vi "FTW-Test-JSON-TypeCoerce-Numbers.vi"() -> (0 "Test Result":errorcluster)   [LabVIEW 2015]
uses:
  src/json/FTW-JSON-Type.ctl
  src/json/core/FTW-JSON-Core-Type.ctl
  src/reflection/FTW-Reflection-Types.ctl
  lib/FTW-KernelFilepath.vi
  codegen/xnode/json/fetch/FTW-JSON-Core-GetFlattenedValue.vi
  src/json/core/FTW-JSON-Core-LibraryReturnValue.vi
  src/error/FTW-ERR-ThrowInvalidReferenceError.vi
  src/json/core/FTW-JSON-Core-ElementType.vi
  codegen/xnode/FTW-JSON-Fetch.xnode
  src/core/type/FTW-Type-JSON.ctl
panel:
  out "JSON String (UTF-8)":string
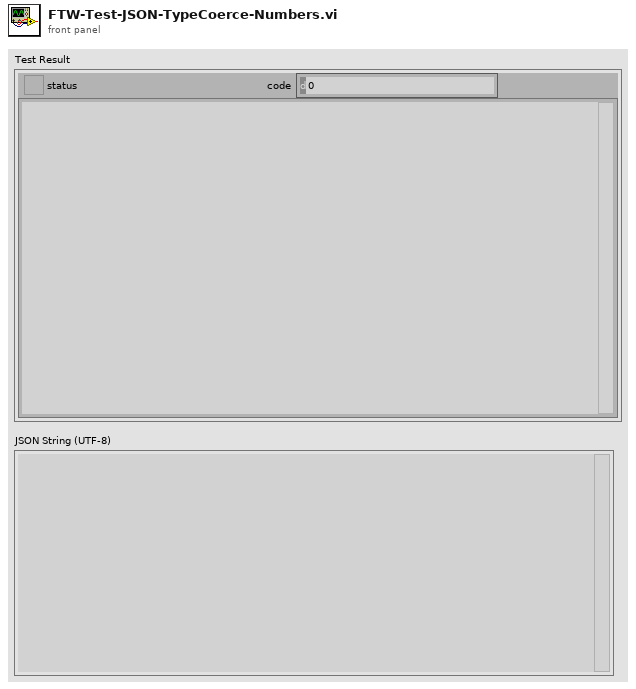
[diagram p1: front panel]
types:
  T1 = typedef "FTW-JSON-Type.ctl" = enum8{"Not Found", "Object", "Array", "String", "Number", "Boolean", "null"}
  T2 = cluster{"Float":ext, "Float":csg, "Float":cdb, "Float":cxt, "Array":ext, "Array":csg, "Array":cdb, "Array":cxt, "NotAKey":ext, "NotAKey":csg, "NotAKey":cdb, "NotAKey":cxt}
  T3 = cluster{"Value":cluster{"SGL":sgl, "DBL":dbl}, "Assertion":string}[]
  T4 = cluster{"Value":cluster{"U8":u8, "U16":u16, "U32":u32, "U64":u64, "I8":i8, "I16":i16, "I32":i32, "I64":i64}, "Assertion":string}[]
  T5 = typedef "FTW-Type-JSON.ctl" = refnum<data-value>
  T6 = cluster{"Integer":u8, "Integer":u16, "Integer":u32, "Integer":u64, "Integer":i8, "Integer":i16, "Integer":i32, "Integer":i64}
  T7 = typedef "FTW-JSON-Core-Type.ctl" = enum8{"Object", "Array", "String", "Integer", "Floating Point", "true", "false", "null", "undefined"}
  T8 = cluster{"Float":u8, "Float":u16, "Float":u32, "Float":u64, "Float":i8, "Float":i16, "Float":i32, "Float":i64}
  T9 = cluster{"String":u8, "String":u16, "String":u32, "String":u64, "String":i8, "String":i16, "String":i32, "String":i64}
  T10 = cluster{"BoolTrue":u8, "BoolTrue":u16, "BoolTrue":u32, "BoolTrue":u64, "BoolTrue":i8, "BoolTrue":i16, "BoolTrue":i32, "BoolTrue":i64}
  T11 = cluster{"BoolFalse":u8, "BoolFalse":u16, "BoolFalse":u32, "BoolFalse":u64, "BoolFalse":i8, "BoolFalse":i16, "BoolFalse":i32, "BoolFalse":i64}
  T12 = cluster{"Object":u8, "Object":u16, "Object":u32, "Object":u64, "Object":i8, "Object":i16, "Object":i32, "Object":i64}
  T13 = cluster{"Array":u8, "Array":u16, "Array":u32, "Array":u64, "Array":i8, "Array":i16, "Array":i32, "Array":i64}
  T14 = cluster{"NULL":u8, "NULL":u16, "NULL":u32, "NULL":u64, "NULL":i8, "NULL":i16, "NULL":i32, "NULL":i64}
  T15 = cluster{"NotAKey":u8, "NotAKey":u16, "NotAKey":u32, "NotAKey":u64, "NotAKey":i8, "NotAKey":i16, "NotAKey":i32, "NotAKey":i64}
  T16 = cluster{"U8":u8, "U16":u16, "U32":u32, "U64":u64, "I8":i8, "I16":i16, "I32":i32, "I64":i64}
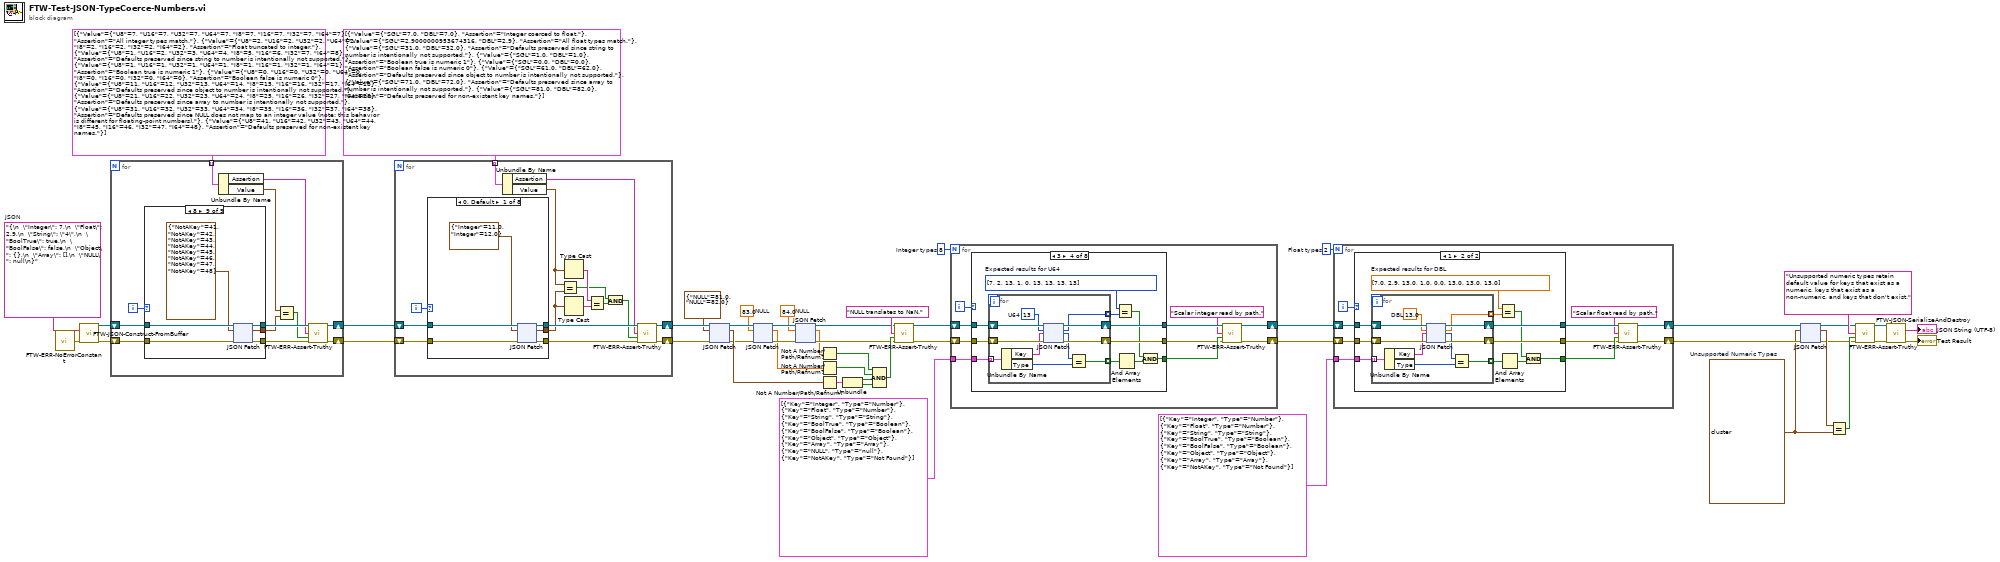
[diagram p0: block diagram]
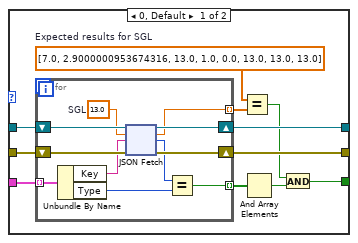
[diagram p2: hidden frame]
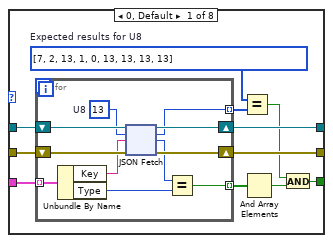
[diagram p3: hidden frame]
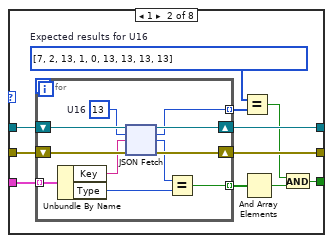
[diagram p4: hidden frame]
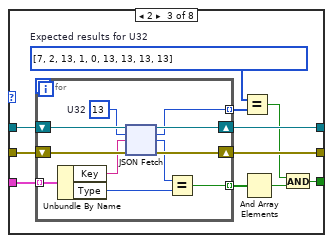
[diagram p5: hidden frame]
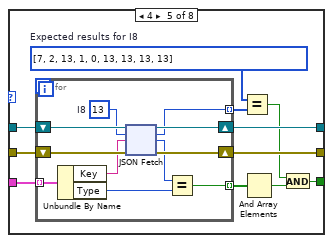
[diagram p6: hidden frame]
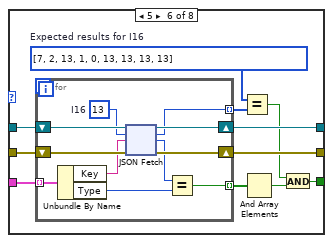
[diagram p7: hidden frame]
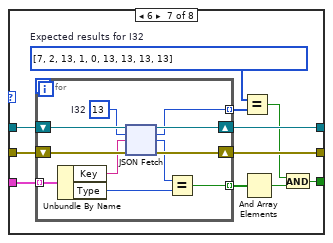
[diagram p8: hidden frame]
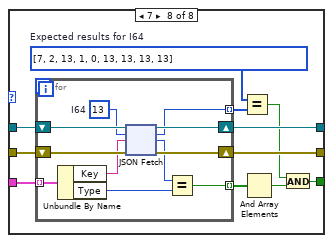
[diagram p9: hidden frame]
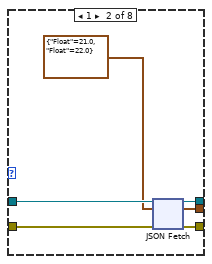
[diagram p10: hidden frame]
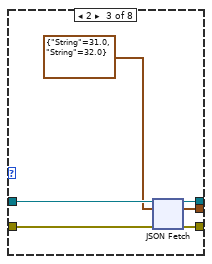
[diagram p11: hidden frame]
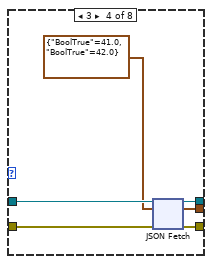
[diagram p12: hidden frame]
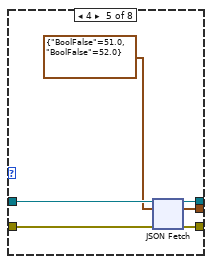
[diagram p13: hidden frame]
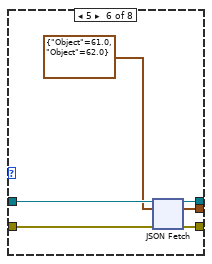
[diagram p14: hidden frame]
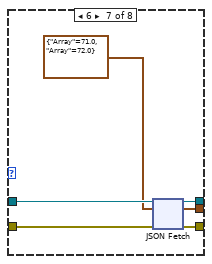
[diagram p15: hidden frame]
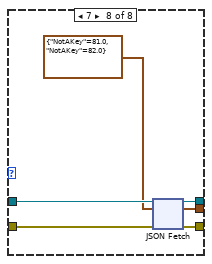
[diagram p16: hidden frame]
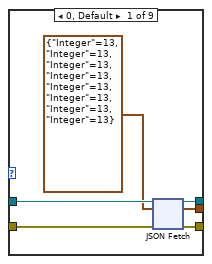
[diagram p17: hidden frame]
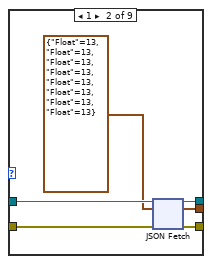
[diagram p18: hidden frame]
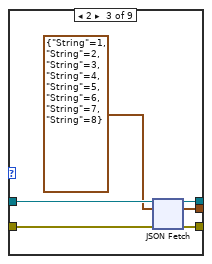
[diagram p19: hidden frame]
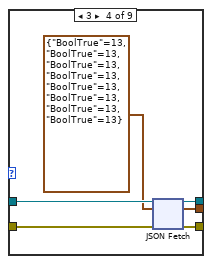
[diagram p20: hidden frame]
diagram:
  w3 = 2  # Float types
  w12 = 84.0  # NULL
  w13 = sgl 83.0  # NULL
  w23 = 8  # Integer types
  w1 = T2 {"Float"=91.0, "Float"=92.0+93.0i, "Float"=94.0+95.0i, "Float"=96.0+97.0i, "Array"=81.0, "Array"=82.0+83.0i, "Array"=84.0+85.0i, "Array"=86.0+87.0i, "NotAKey"=71.0, "NotAKey"=72.0+73.0i, "NotAKey"=74.0+75.0i, "NotAKey"=76.0+77.0i}  # Unsupported Numeric Types
  w45 = "{\n  \"Integer\": 7,\n  \"Float\": 2.9,\n  \"String\": \"4\",\n  \"BoolTrue\": true,\n  \"BoolFalse\": false,\n  \"Object\": {},\n  \"Array\": [],\n  \"NULL\": null\n}"  # JSON
  n1 = call "FTW-ERR-NoErrorConstant.vi"() -> ("no error"=w44:errorcluster)
  n2 = call "FTW-JSON-Construct-FromBuffer.vi"("JSON String (UTF-8)"=w45, "error in"=w44) -> ("JSON"=w42:T5, "error out"=w43:errorcluster)  [unwired: 12 in]
  n3 = for {
    shift-right: [w53] -> w39
    shift-left: w43 -> [w58]
    shift-right: [w56] -> w40
    shift-left: w42 -> [w57]
    tunnel: T4 [{"Value"={"U8"=7, "U16"=7, "U32"=7, "U64"=7, "I8"=7, "I16"=7, "I32"=7, "I64"=7}, "Assertion"="All integer types match."}, {"Value"={"U8"=2, "U16"=2, "U32"=2, "U64"=2, "I8"=2, "I16"=2, "I32"=2, "I64"=2}, "Assertion"="Float truncated to integer."}, {"Value"={"U8"=1, "U16"=2, "U32"=3, "U64"=4, "I8"=5, "I16"=6, "I32"=7, "I64"=8}, "Assertion"="Defaults preserved since string to number is intentionally not supported."}, {"Value"={"U8"=1, "U16"=1, "U32"=1, "U64"=1, "I8"=1, "I16"=1, "I32"=1, "I64"=1}, "Assertion"="Boolean true is numeric 1"}, {"Value"={"U8"=0, "U16"=0, "U32"=0, "U64"=0, "I8"=0, "I16"=0, "I32"=0, "I64"=0}, "Assertion"="Boolean false is numeric 0"}, {"Value"={"U8"=11, "U16"=12, "U32"=13, "U64"=14, "I8"=15, "I16"=16, "I32"=17, "I64"=18}, "Assertion"="Defaults preserved since object to number is intentionally not supported."}, {"Value"={"U8"=21, "U16"=22, "U32"=23, "U64"=24, "I8"=25, "I16"=26, "I32"=27, "I64"=28}, "Assertion"="Defaults preserved since array to number is intentionally not supported."}, {"Value"={"U8"=31, "U16"=32, "U32"=33, "U64"=34, "I8"=35, "I16"=36, "I32"=37, "I64"=38}, "Assertion"="Defaults preserved since NULL does not map to an integer value (note: this behavior is different for floating-point numbers)."}, {"Value"={"U8"=41, "U16"=42, "U32"=43, "U64"=44, "I8"=45, "I16"=46, "I32"=47, "I64"=48}, "Assertion"="Defaults preserved for non-existent key names."}] -> [w54] mode=indexing
    i -> [w55]
    n4 = case shown="8" w55 {
      tunnel: w58 -> [w64 w123 w182 w241 w300 w359 w418 w477 w536]
      tunnel: w57 -> [w63 w122 w181 w240 w299 w358 w417 w476 w535]
      tunnel: [w61 w120 w179 w238 w297 w356 w415 w474 w533] -> w56
      tunnel: [w60 w119 w178 w237 w296 w355 w414 w473 w532] -> w52
      tunnel: [w59 w118 w177 w236 w295 w354 w413 w472 w531] -> w50
      frame 0, Default {
        n5 = xnode "JSON Fetch"("JSON"=w63, "Element Type and Default Value"=T6 {"Integer"=13, "Integer"=13, "Integer"=13, "Integer"=13, "Integer"=13, "Integer"=13, "Integer"=13, "Integer"=13}, "error in"=w64) -> ("JSON out"=w61:T5, "Value"=w59:T6, "error out"=w60:errorcluster)  [unwired: 2 in, 1 out]
      }
      frame 1 {
        n6 = xnode "JSON Fetch"("JSON"=w122, "Element Type and Default Value"=T8 {"Float"=13, "Float"=13, "Float"=13, "Float"=13, "Float"=13, "Float"=13, "Float"=13, "Float"=13}, "error in"=w123) -> ("JSON out"=w120:T5, "Value"=w118:T8, "error out"=w119:errorcluster)  [unwired: 2 in, 1 out]
      }
      frame 2 {
        n7 = xnode "JSON Fetch"("JSON"=w181, "Element Type and Default Value"=T9 {"String"=1, "String"=2, "String"=3, "String"=4, "String"=5, "String"=6, "String"=7, "String"=8}, "error in"=w182) -> ("JSON out"=w179:T5, "Value"=w177:T9, "error out"=w178:errorcluster)  [unwired: 2 in, 1 out]
      }
      frame 3 {
        n8 = xnode "JSON Fetch"("JSON"=w240, "Element Type and Default Value"=T10 {"BoolTrue"=13, "BoolTrue"=13, "BoolTrue"=13, "BoolTrue"=13, "BoolTrue"=13, "BoolTrue"=13, "BoolTrue"=13, "BoolTrue"=13}, "error in"=w241) -> ("JSON out"=w238:T5, "Value"=w236:T10, "error out"=w237:errorcluster)  [unwired: 2 in, 1 out]
      }
      frame 4 {
        n9 = xnode "JSON Fetch"("JSON"=w299, "Element Type and Default Value"=T11 {"BoolFalse"=13, "BoolFalse"=13, "BoolFalse"=13, "BoolFalse"=13, "BoolFalse"=13, "BoolFalse"=13, "BoolFalse"=13, "BoolFalse"=13}, "error in"=w300) -> ("JSON out"=w297:T5, "Value"=w295:T11, "error out"=w296:errorcluster)  [unwired: 2 in, 1 out]
      }
      frame 5 {
        n10 = xnode "JSON Fetch"("JSON"=w358, "Element Type and Default Value"=T12 {"Object"=11, "Object"=12, "Object"=13, "Object"=14, "Object"=15, "Object"=16, "Object"=17, "Object"=18}, "error in"=w359) -> ("JSON out"=w356:T5, "Value"=w354:T12, "error out"=w355:errorcluster)  [unwired: 2 in, 1 out]
      }
      frame 6 {
        n11 = xnode "JSON Fetch"("JSON"=w417, "Element Type and Default Value"=T13 {"Array"=21, "Array"=22, "Array"=23, "Array"=24, "Array"=25, "Array"=26, "Array"=27, "Array"=28}, "error in"=w418) -> ("JSON out"=w415:T5, "Value"=w413:T13, "error out"=w414:errorcluster)  [unwired: 2 in, 1 out]
      }
      frame 7 {
        n12 = xnode "JSON Fetch"("JSON"=w476, "Element Type and Default Value"=T14 {"NULL"=31, "NULL"=32, "NULL"=33, "NULL"=34, "NULL"=35, "NULL"=36, "NULL"=37, "NULL"=38}, "error in"=w477) -> ("JSON out"=w474:T5, "Value"=w472:T14, "error out"=w473:errorcluster)  [unwired: 2 in, 1 out]
      }
      frame 8 {
        n13 = xnode "JSON Fetch"("JSON"=w535, "Element Type and Default Value"=T15 {"NotAKey"=41, "NotAKey"=42, "NotAKey"=43, "NotAKey"=44, "NotAKey"=45, "NotAKey"=46, "NotAKey"=47, "NotAKey"=48}, "error in"=w536) -> ("JSON out"=w533:T5, "Value"=w531:T15, "error out"=w532:errorcluster)  [unwired: 2 in, 1 out]
      }
    }
    n14 = Unbundle By Name(w54) -> ("Assertion"=w51:string, "Value"=w49:T16)
    n15 = Equal?(x=w49, y=w50) -> (x = y?=w48:bool)
    n16 = call "FTW-ERR-Assert-Truthy.vi"("Assertion"=w51, "Assertion holds true?"=w48, "error in"=w52) -> ("error out"=w53:errorcluster)  [unwired: 12 in]
  }
  n17 = for {
    shift-right: [w599] -> w36
    shift-left: w39 -> [w604]
    shift-right: [w602] -> w37
    shift-left: w40 -> [w603]
    tunnel: T3 [{"Value"={"SGL"=7.0, "DBL"=7.0}, "Assertion"="Integer coerced to float."}, {"Value"={"SGL"=2.9, "DBL"=2.9}, "Assertion"="All float types match."}, {"Value"={"SGL"=31.0, "DBL"=32.0}, "Assertion"="Defaults preserved since string to number is intentionally not supported."}, {"Value"={"SGL"=1.0, "DBL"=1.0}, "Assertion"="Boolean true is numeric 1"}, {"Value"={"SGL"=0.0, "DBL"=0.0}, "Assertion"="Boolean false is numeric 0"}, {"Value"={"SGL"=61.0, "DBL"=62.0}, "Assertion"="Defaults preserved since object to number is intentionally not supported."}, {"Value"={"SGL"=71.0, "DBL"=72.0}, "Assertion"="Defaults preserved since array to number is intentionally not supported."}, {"Value"={"SGL"=81.0, "DBL"=82.0}, "Assertion"="Defaults preserved for non-existent key names."}] -> [w600] mode=indexing
    i -> [w601]
    n18 = case shown="0, Default" w601 {
      tunnel: w604 -> [w610 w669 w728 w787 w846 w905 w964 w1023]
      tunnel: w603 -> [w609 w668 w727 w786 w845 w904 w963 w1022]
      tunnel: [w607 w666 w725 w784 w843 w902 w961 w1020] -> w602
      tunnel: [w606 w665 w724 w783 w842 w901 w960 w1019] -> w598
      tunnel: [w605 w664 w723 w782 w841 w900 w959 w1018] -> w595
      frame 0, Default {
        n19 = xnode "JSON Fetch"("JSON"=w609, "Element Type and Default Value"=cluster{"Integer":sgl, "Integer":dbl} {"Integer"=11.0, "Integer"=12.0}, "error in"=w610) -> ("JSON out"=w607:T5, "Value"=w605:cluster{"Integer":sgl, "Integer":dbl}, "error out"=w606:errorcluster)  [unwired: 2 in, 1 out]
      }
      frame 1 {
        n20 = xnode "JSON Fetch"("JSON"=w668, "Element Type and Default Value"=cluster{"Float":sgl, "Float":dbl} {"Float"=21.0, "Float"=22.0}, "error in"=w669) -> ("JSON out"=w666:T5, "Value"=w664:cluster{"Float":sgl, "Float":dbl}, "error out"=w665:errorcluster)  [unwired: 2 in, 1 out]
      }
      frame 2 {
        n21 = xnode "JSON Fetch"("JSON"=w727, "Element Type and Default Value"=cluster{"String":sgl, "String":dbl} {"String"=31.0, "String"=32.0}, "error in"=w728) -> ("JSON out"=w725:T5, "Value"=w723:cluster{"String":sgl, "String":dbl}, "error out"=w724:errorcluster)  [unwired: 2 in, 1 out]
      }
      frame 3 {
        n22 = xnode "JSON Fetch"("JSON"=w786, "Element Type and Default Value"=cluster{"BoolTrue":sgl, "BoolTrue":dbl} {"BoolTrue"=41.0, "BoolTrue"=42.0}, "error in"=w787) -> ("JSON out"=w784:T5, "Value"=w782:cluster{"BoolTrue":sgl, "BoolTrue":dbl}, "error out"=w783:errorcluster)  [unwired: 2 in, 1 out]
      }
      frame 4 {
        n23 = xnode "JSON Fetch"("JSON"=w845, "Element Type and Default Value"=cluster{"BoolFalse":sgl, "BoolFalse":dbl} {"BoolFalse"=51.0, "BoolFalse"=52.0}, "error in"=w846) -> ("JSON out"=w843:T5, "Value"=w841:cluster{"BoolFalse":sgl, "BoolFalse":dbl}, "error out"=w842:errorcluster)  [unwired: 2 in, 1 out]
      }
      frame 5 {
        n24 = xnode "JSON Fetch"("JSON"=w904, "Element Type and Default Value"=cluster{"Object":sgl, "Object":dbl} {"Object"=61.0, "Object"=62.0}, "error in"=w905) -> ("JSON out"=w902:T5, "Value"=w900:cluster{"Object":sgl, "Object":dbl}, "error out"=w901:errorcluster)  [unwired: 2 in, 1 out]
      }
      frame 6 {
        n25 = xnode "JSON Fetch"("JSON"=w963, "Element Type and Default Value"=cluster{"Array":sgl, "Array":dbl} {"Array"=71.0, "Array"=72.0}, "error in"=w964) -> ("JSON out"=w961:T5, "Value"=w959:cluster{"Array":sgl, "Array":dbl}, "error out"=w960:errorcluster)  [unwired: 2 in, 1 out]
      }
      frame 7 {
        n26 = xnode "JSON Fetch"("JSON"=w1022, "Element Type and Default Value"=cluster{"NotAKey":sgl, "NotAKey":dbl} {"NotAKey"=81.0, "NotAKey"=82.0}, "error in"=w1023) -> ("JSON out"=w1020:T5, "Value"=w1018:cluster{"NotAKey":sgl, "NotAKey":dbl}, "error out"=w1019:errorcluster)  [unwired: 2 in, 1 out]
      }
    }
    n27 = Unbundle By Name(w600) -> ("Assertion"=w597:string, "Value"=w596:cluster{"SGL":sgl, "DBL":dbl})
    n28 = Equal?(x=w596, y=w595) -> (x = y?=w592:bool)
    n29 = Type Cast(x=w596) -> (*(type *) &x=w594:string)  [unwired: 1 in]
    n30 = Type Cast(x=w595) -> (*(type *) &x=w593:string)  [unwired: 1 in]
    n31 = Equal?(x=w594, y=w593) -> (x = y?=w591:bool)
    n32 = And(x=w592, y=w591) -> (x .and. y?=w590:bool)
    n33 = call "FTW-ERR-Assert-Truthy.vi"("Assertion"=w597, "Assertion holds true?"=w590, "error in"=w598) -> ("error out"=w599:errorcluster)  [unwired: 12 in]
  }
  n34 = xnode "JSON Fetch"("JSON"=w37, "Element Type and Default Value"=cluster{"NULL":sgl, "NULL":dbl} {"NULL"=81.0, "NULL"=82.0}, "error in"=w36) -> ("JSON out"=w20:T5, "Value"=w34:cluster{"NULL":sgl, "NULL":dbl}, "error out"=w16:errorcluster)  [unwired: 2 in, 1 out]
  n35 = xnode "JSON Fetch"("JSON"=w20, "Element Type and Default Value"=w13, "error in"=w16) -> ("JSON out"=w19:T5, "Value"=w11:sgl, "error out"=w15:errorcluster)  [unwired: 2 in, 1 out]
  n36 = xnode "JSON Fetch"("JSON"=w19, "Element Type and Default Value"=w12, "error in"=w15) -> ("JSON out"=w18:T5, "Value"=w10:dbl, "error out"=w17:errorcluster)  [unwired: 2 in, 1 out]
  n37 = Not A Number/Path/Refnum?(number/path/refnum=w10) -> (NaN/Path/Refnum?=w8:bool)
  n38 = Not A Number/Path/Refnum?(number/path/refnum=w11) -> (NaN/Path/Refnum?=w9:bool)
  n39 = Not A Number/Path/Refnum?(number/path/refnum=w34) -> (NaN/Path/Refnum?=w33:cluster{"NULL":bool, "NULL":bool})
  n40 = Unbundle(w33) -> ("NULL"=w32:bool, "NULL"=w31:bool)
  n41 = Compound Arithmetic op=AND(w8, w9, w32, w31) -> (w30:bool)
  n42 = call "FTW-ERR-Assert-Truthy.vi"("Assertion"="NULL translates to NaN.", "Assertion holds true?"=w30, "error in"=w17) -> ("error out"=w14:errorcluster)  [unwired: 12 in]
  n43 = for {
    N: w23 -> [_]
    tunnel: cluster{"Key":string, "Type":T1}[] [{"Key"="Integer", "Type"=enum."Number"}, {"Key"="Float", "Type"=enum."Number"}, {"Key"="String", "Type"=enum."String"}, {"Key"="BoolTrue", "Type"=enum."Boolean"}, {"Key"="BoolFalse", "Type"=enum."Boolean"}, {"Key"="Object", "Type"=enum."Object"}, {"Key"="Array", "Type"=enum."Array"}, {"Key"="NULL", "Type"=enum."null"}, {"Key"="NotAKey", "Type"=enum."Not Found"}] -> [w1082]
    shift-right: [w1084] -> w7
    shift-left: w18 -> [w1085]
    shift-right: [w1078] -> w6
    shift-left: w14 -> [w1083]
    i -> [w1081]
    n44 = case shown="3" w1081 {
      tunnel: w1085 -> [w1096 w1162 w1228 w1294 w1360 w1426 w1492 w1558]
      tunnel: [w1095 w1161 w1227 w1293 w1359 w1425 w1491 w1557] -> w1084
      tunnel: w1083 -> [w1094 w1160 w1226 w1292 w1358 w1424 w1490 w1556]
      tunnel: [w1091 w1157 w1223 w1289 w1355 w1421 w1487 w1553] -> w1077
      tunnel: w1082 -> [w1090 w1156 w1222 w1288 w1354 w1420 w1486 w1552]
      tunnel: [w1086 w1152 w1218 w1284 w1350 w1416 w1482 w1548] -> w1079
      frame 0, Default {
        w1092 = u8[] [7, 2, 13, 1, 0, 13, 13, 13, 13]  # Expected results for U8
        n45 = for {
          shift-right: [w1104] -> w1095
          shift-left: w1096 -> [w1107]
          shift-right: [w1105] -> w1091
          shift-left: w1094 -> [w1106]
          tunnel: [w1102] -> w1093 mode=indexing
          tunnel: w1090 -> [w1100] mode=indexing
          tunnel: [w1097] -> w1089 mode=indexing
          w1103 = u8 13  # U8
          n46 = Unbundle By Name(w1100) -> ("Key"=w1099:string, "Type"=w1098:T1)
          n47 = xnode "JSON Fetch"("JSON"=w1107, "Element Type and Default Value"=w1103, "Element Path"=w1099, "error in"=w1106) -> ("JSON out"=w1104:T5, "Value"=w1102:u8, "JSON Element Type"=w1101:T1, "error out"=w1105:errorcluster)  [unwired: 1 in]
          n48 = Equal?(x=w1101, y=w1098) -> (x = y?=w1097:bool)
        }
        n49 = Equal?(x=w1092, y=w1093) -> (x = y?=w1088:bool)
        n50 = And Array Elements(Boolean array=w1089) -> (logical AND=w1087:bool)
        n51 = And(x=w1088, y=w1087) -> (x .and. y?=w1086:bool)
      }
      frame 1 {
        w1158 = u16[] [7, 2, 13, 1, 0, 13, 13, 13, 13]  # Expected results for U16
        n52 = for {
          shift-right: [w1170] -> w1161
          shift-left: w1162 -> [w1173]
          shift-right: [w1171] -> w1157
          shift-left: w1160 -> [w1172]
          tunnel: [w1168] -> w1159 mode=indexing
          tunnel: w1156 -> [w1166] mode=indexing
          tunnel: [w1163] -> w1155 mode=indexing
          w1169 = u16 13  # U16
          n53 = Unbundle By Name(w1166) -> ("Key"=w1165:string, "Type"=w1164:T1)
          n54 = xnode "JSON Fetch"("JSON"=w1173, "Element Type and Default Value"=w1169, "Element Path"=w1165, "error in"=w1172) -> ("JSON out"=w1170:T5, "Value"=w1168:u16, "JSON Element Type"=w1167:T1, "error out"=w1171:errorcluster)  [unwired: 1 in]
          n55 = Equal?(x=w1167, y=w1164) -> (x = y?=w1163:bool)
        }
        n56 = Equal?(x=w1158, y=w1159) -> (x = y?=w1154:bool)
        n57 = And Array Elements(Boolean array=w1155) -> (logical AND=w1153:bool)
        n58 = And(x=w1154, y=w1153) -> (x .and. y?=w1152:bool)
      }
      frame 2 {
        w1224 = u32[] [7, 2, 13, 1, 0, 13, 13, 13, 13]  # Expected results for U32
        n59 = for {
          shift-right: [w1236] -> w1227
          shift-left: w1228 -> [w1239]
          shift-right: [w1237] -> w1223
          shift-left: w1226 -> [w1238]
          tunnel: [w1234] -> w1225 mode=indexing
          tunnel: w1222 -> [w1232] mode=indexing
          tunnel: [w1229] -> w1221 mode=indexing
          w1235 = u32 13  # U32
          n60 = Unbundle By Name(w1232) -> ("Key"=w1231:string, "Type"=w1230:T1)
          n61 = xnode "JSON Fetch"("JSON"=w1239, "Element Type and Default Value"=w1235, "Element Path"=w1231, "error in"=w1238) -> ("JSON out"=w1236:T5, "Value"=w1234:u32, "JSON Element Type"=w1233:T1, "error out"=w1237:errorcluster)  [unwired: 1 in]
          n62 = Equal?(x=w1233, y=w1230) -> (x = y?=w1229:bool)
        }
        n63 = Equal?(x=w1224, y=w1225) -> (x = y?=w1220:bool)
        n64 = And Array Elements(Boolean array=w1221) -> (logical AND=w1219:bool)
        n65 = And(x=w1220, y=w1219) -> (x .and. y?=w1218:bool)
      }
      frame 3 {
        w1290 = u64[] [7, 2, 13, 1, 0, 13, 13, 13, 13]  # Expected results for U64
        n66 = for {
          shift-right: [w1302] -> w1293
          shift-left: w1294 -> [w1305]
          shift-right: [w1303] -> w1289
          shift-left: w1292 -> [w1304]
          tunnel: [w1300] -> w1291 mode=indexing
          tunnel: w1288 -> [w1298] mode=indexing
          tunnel: [w1295] -> w1287 mode=indexing
          w1301 = u64 13  # U64
          n67 = Unbundle By Name(w1298) -> ("Key"=w1297:string, "Type"=w1296:T1)
          n68 = xnode "JSON Fetch"("JSON"=w1305, "Element Type and Default Value"=w1301, "Element Path"=w1297, "error in"=w1304) -> ("JSON out"=w1302:T5, "Value"=w1300:u64, "JSON Element Type"=w1299:T1, "error out"=w1303:errorcluster)  [unwired: 1 in]
          n69 = Equal?(x=w1299, y=w1296) -> (x = y?=w1295:bool)
        }
        n70 = Equal?(x=w1290, y=w1291) -> (x = y?=w1286:bool)
        n71 = And Array Elements(Boolean array=w1287) -> (logical AND=w1285:bool)
        n72 = And(x=w1286, y=w1285) -> (x .and. y?=w1284:bool)
      }
      frame 4 {
        w1356 = i8[] [7, 2, 13, 1, 0, 13, 13, 13, 13]  # Expected results for I8
        n73 = for {
          shift-right: [w1368] -> w1359
          shift-left: w1360 -> [w1371]
          shift-right: [w1369] -> w1355
          shift-left: w1358 -> [w1370]
          tunnel: [w1366] -> w1357 mode=indexing
          tunnel: w1354 -> [w1364] mode=indexing
          tunnel: [w1361] -> w1353 mode=indexing
          w1367 = i8 13  # I8
          n74 = Unbundle By Name(w1364) -> ("Key"=w1363:string, "Type"=w1362:T1)
          n75 = xnode "JSON Fetch"("JSON"=w1371, "Element Type and Default Value"=w1367, "Element Path"=w1363, "error in"=w1370) -> ("JSON out"=w1368:T5, "Value"=w1366:i8, "JSON Element Type"=w1365:T1, "error out"=w1369:errorcluster)  [unwired: 1 in]
          n76 = Equal?(x=w1365, y=w1362) -> (x = y?=w1361:bool)
        }
        n77 = Equal?(x=w1356, y=w1357) -> (x = y?=w1352:bool)
        n78 = And Array Elements(Boolean array=w1353) -> (logical AND=w1351:bool)
        n79 = And(x=w1352, y=w1351) -> (x .and. y?=w1350:bool)
      }
      frame 5 {
        w1422 = i16[] [7, 2, 13, 1, 0, 13, 13, 13, 13]  # Expected results for I16
        n80 = for {
          shift-right: [w1434] -> w1425
          shift-left: w1426 -> [w1437]
          shift-right: [w1435] -> w1421
          shift-left: w1424 -> [w1436]
          tunnel: [w1432] -> w1423 mode=indexing
          tunnel: w1420 -> [w1430] mode=indexing
          tunnel: [w1427] -> w1419 mode=indexing
          w1433 = i16 13  # I16
          n81 = Unbundle By Name(w1430) -> ("Key"=w1429:string, "Type"=w1428:T1)
          n82 = xnode "JSON Fetch"("JSON"=w1437, "Element Type and Default Value"=w1433, "Element Path"=w1429, "error in"=w1436) -> ("JSON out"=w1434:T5, "Value"=w1432:i16, "JSON Element Type"=w1431:T1, "error out"=w1435:errorcluster)  [unwired: 1 in]
          n83 = Equal?(x=w1431, y=w1428) -> (x = y?=w1427:bool)
        }
        n84 = Equal?(x=w1422, y=w1423) -> (x = y?=w1418:bool)
        n85 = And Array Elements(Boolean array=w1419) -> (logical AND=w1417:bool)
        n86 = And(x=w1418, y=w1417) -> (x .and. y?=w1416:bool)
      }
      frame 6 {
        w1488 = i32[] [7, 2, 13, 1, 0, 13, 13, 13, 13]  # Expected results for I32
        n87 = for {
          shift-right: [w1500] -> w1491
          shift-left: w1492 -> [w1503]
          shift-right: [w1501] -> w1487
          shift-left: w1490 -> [w1502]
          tunnel: [w1498] -> w1489 mode=indexing
          tunnel: w1486 -> [w1496] mode=indexing
          tunnel: [w1493] -> w1485 mode=indexing
          w1499 = 13  # I32
          n88 = Unbundle By Name(w1496) -> ("Key"=w1495:string, "Type"=w1494:T1)
          n89 = xnode "JSON Fetch"("JSON"=w1503, "Element Type and Default Value"=w1499, "Element Path"=w1495, "error in"=w1502) -> ("JSON out"=w1500:T5, "Value"=w1498:i32, "JSON Element Type"=w1497:T1, "error out"=w1501:errorcluster)  [unwired: 1 in]
          n90 = Equal?(x=w1497, y=w1494) -> (x = y?=w1493:bool)
        }
        n91 = Equal?(x=w1488, y=w1489) -> (x = y?=w1484:bool)
        n92 = And Array Elements(Boolean array=w1485) -> (logical AND=w1483:bool)
        n93 = And(x=w1484, y=w1483) -> (x .and. y?=w1482:bool)
      }
      frame 7 {
        w1554 = i64[] [7, 2, 13, 1, 0, 13, 13, 13, 13]  # Expected results for I64
        n94 = for {
          shift-right: [w1566] -> w1557
          shift-left: w1558 -> [w1569]
          shift-right: [w1567] -> w1553
          shift-left: w1556 -> [w1568]
          tunnel: [w1564] -> w1555 mode=indexing
          tunnel: w1552 -> [w1562] mode=indexing
          tunnel: [w1559] -> w1551 mode=indexing
          w1565 = i64 13  # I64
          n95 = Unbundle By Name(w1562) -> ("Key"=w1561:string, "Type"=w1560:T1)
          n96 = xnode "JSON Fetch"("JSON"=w1569, "Element Type and Default Value"=w1565, "Element Path"=w1561, "error in"=w1568) -> ("JSON out"=w1566:T5, "Value"=w1564:i64, "JSON Element Type"=w1563:T1, "error out"=w1567:errorcluster)  [unwired: 1 in]
          n97 = Equal?(x=w1563, y=w1560) -> (x = y?=w1559:bool)
        }
        n98 = Equal?(x=w1554, y=w1555) -> (x = y?=w1550:bool)
        n99 = And Array Elements(Boolean array=w1551) -> (logical AND=w1549:bool)
        n100 = And(x=w1550, y=w1549) -> (x .and. y?=w1548:bool)
      }
    }
    n101 = call "FTW-ERR-Assert-Truthy.vi"("Assertion"="Scalar integer read by path.", "Assertion holds true?"=w1079, "error in"=w1077) -> ("error out"=w1078:errorcluster)  [unwired: 12 in]
  }
  n102 = for {
    N: w3 -> [_]
    tunnel: cluster{"Key":string, "Type":T1}[] [{"Key"="Integer", "Type"=enum."Number"}, {"Key"="Float", "Type"=enum."Number"}, {"Key"="String", "Type"=enum."String"}, {"Key"="BoolTrue", "Type"=enum."Boolean"}, {"Key"="BoolFalse", "Type"=enum."Boolean"}, {"Key"="Object", "Type"=enum."Object"}, {"Key"="Array", "Type"=enum."Array"}, {"Key"="NotAKey", "Type"=enum."Not Found"}] -> [w1619]
    shift-right: [w1621] -> w4
    shift-left: w7 -> [w1622]
    shift-right: [w1615] -> w5
    shift-left: w6 -> [w1620]
    i -> [w1618]
    n103 = case shown="1" w1618 {
      tunnel: w1622 -> [w1633 w1699]
      tunnel: [w1632 w1698] -> w1621
      tunnel: w1620 -> [w1631 w1697]
      tunnel: [w1628 w1694] -> w1614
      tunnel: w1619 -> [w1627 w1693]
      tunnel: [w1623 w1689] -> w1616
      frame 0, Default {
        w1629 = sgl[] [7.0, 2.9, 13.0, 1.0, 0.0, 13.0, 13.0, 13.0]  # Expected results for SGL
        n104 = for {
          shift-right: [w1641] -> w1632
          shift-left: w1633 -> [w1644]
          shift-right: [w1642] -> w1628
          shift-left: w1631 -> [w1643]
          tunnel: [w1639] -> w1630 mode=indexing
          tunnel: w1627 -> [w1637] mode=indexing
          tunnel: [w1634] -> w1626 mode=indexing
          w1640 = sgl 13.0  # SGL
          n105 = Unbundle By Name(w1637) -> ("Key"=w1636:string, "Type"=w1635:T1)
          n106 = xnode "JSON Fetch"("JSON"=w1644, "Element Type and Default Value"=w1640, "Element Path"=w1636, "error in"=w1643) -> ("JSON out"=w1641:T5, "Value"=w1639:sgl, "JSON Element Type"=w1638:T1, "error out"=w1642:errorcluster)  [unwired: 1 in]
          n107 = Equal?(x=w1638, y=w1635) -> (x = y?=w1634:bool)
        }
        n108 = Equal?(x=w1629, y=w1630) -> (x = y?=w1625:bool)
        n109 = And Array Elements(Boolean array=w1626) -> (logical AND=w1624:bool)
        n110 = And(x=w1625, y=w1624) -> (x .and. y?=w1623:bool)
      }
      frame 1 {
        w1695 = dbl[] [7.0, 2.9, 13.0, 1.0, 0.0, 13.0, 13.0, 13.0]  # Expected results for DBL
        n111 = for {
          shift-right: [w1707] -> w1698
          shift-left: w1699 -> [w1710]
          shift-right: [w1708] -> w1694
          shift-left: w1697 -> [w1709]
          tunnel: [w1705] -> w1696 mode=indexing
          tunnel: w1693 -> [w1703] mode=indexing
          tunnel: [w1700] -> w1692 mode=indexing
          w1706 = 13.0  # DBL
          n112 = Unbundle By Name(w1703) -> ("Key"=w1702:string, "Type"=w1701:T1)
          n113 = xnode "JSON Fetch"("JSON"=w1710, "Element Type and Default Value"=w1706, "Element Path"=w1702, "error in"=w1709) -> ("JSON out"=w1707:T5, "Value"=w1705:dbl, "JSON Element Type"=w1704:T1, "error out"=w1708:errorcluster)  [unwired: 1 in]
          n114 = Equal?(x=w1704, y=w1701) -> (x = y?=w1700:bool)
        }
        n115 = Equal?(x=w1695, y=w1696) -> (x = y?=w1691:bool)
        n116 = And Array Elements(Boolean array=w1692) -> (logical AND=w1690:bool)
        n117 = And(x=w1691, y=w1690) -> (x .and. y?=w1689:bool)
      }
    }
    n118 = call "FTW-ERR-Assert-Truthy.vi"("Assertion"="Scalar float read by path.", "Assertion holds true?"=w1616, "error in"=w1614) -> ("error out"=w1615:errorcluster)  [unwired: 12 in]
  }
  n119 = xnode "JSON Fetch"("JSON"=w4, "Element Type and Default Value"=w1, "error in"=w5) -> ("JSON out"=w21:T5, "Value"=w27:T2, "error out"=w25:errorcluster)  [unwired: 2 in, 1 out]
  n120 = Equal?(x=w27, y=w1) -> (x = y?=w26:bool)
  n121 = call "FTW-ERR-Assert-Truthy.vi"("Assertion"="Unsupported numeric types retain default value for keys that exist as a numeric, keys that exist as a non-numeric, and keys that don't exist.", "Assertion holds true?"=w26, "error in"=w25) -> ("error out"=w22:errorcluster)  [unwired: 12 in]
  n122 = call "FTW-JSON-SerializeAndDestroy.vi"("JSON"=w21, "error in"=w22) -> ("JSON String (UTF-8)"=→"JSON String (UTF-8)":string, "error out"=→"Test Result":errorcluster)  [unwired: 12 in]
